vi "MSEncoder SubVI EndofCase.vi"(10 "error in (no error)":errorcluster, 11 "Case codes":u64[](array[numeric])) -> (2 "error out":errorcluster, 3 "Case codes with end":u64[](array[numeric]))   [LabVIEW 2018, in "MSEncoder.lvclass"]
uses:
  MSEncoder.lvclass
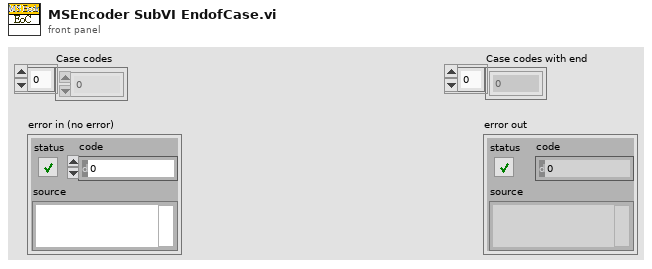
[diagram p1: front panel]
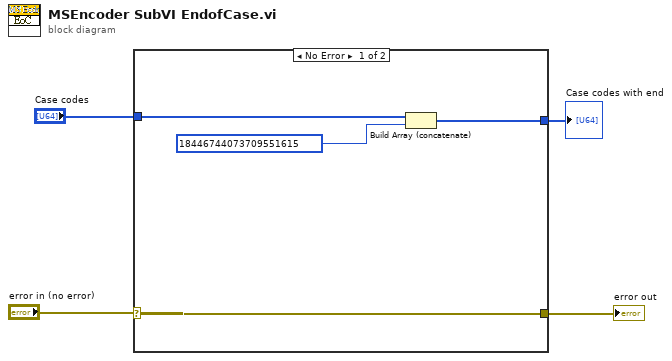
[diagram p0: block diagram]
diagram:
  n1 = case shown="No Error" "error in (no error)" {
    selector: "error in (no error)" -> [w8 w9]
    tunnel: [w8 w9] -> w3
    tunnel: "Case codes" -> [w7 _]
    tunnel: [w6 _] -> w1
    frame No Error {
      n2 = Build Array (concatenate)(w7, u64 18446744073709551615) -> (w6:u64[])
    }
    frame Error {
    }
  }
  "error out" <- w3
  "Case codes with end" <- w1
